vi "Przeliczanie azymutu na kąt i redukcja zakresu stopni.vi"(4 "Azymut [stoponie]":dbl) -> (1 "Kąt [stopnie]":dbl)   [LabVIEW 2012, in "Biblioteka moduł map v3.lvlib" / "Matematyczne.lvlib"]
uses:
  Matematyczne.lvlib
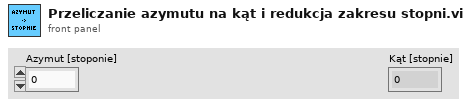
[diagram p1: front panel]
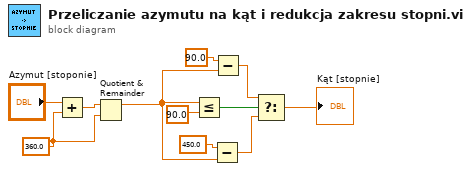
[diagram p0: block diagram]
diagram:
  w4 = 360.0 ("y")
  n1 = Add(x="Azymut [stoponie]", y=w4) -> (x+y=w5:dbl)
  n2 = Quotient & Remainder(x=w5, y=w4) -> (x-y*floor(x/y)=w3:dbl)  [unwired: 1 out]
  n3 = Less Or Equal?(x=w3, y=90.0) -> (x <= y?=w9:bool)
  n4 = Subtract(x=450.0, y=w3) -> (x-y=w8:dbl)
  n5 = Subtract(x=90.0, y=w3) -> (x-y=w6:dbl)
  n6 = Select(t=w6, s=w9, f=w8) -> (s? t:f=→"Kąt [stopnie]":dbl)
